vi "Handle Actor Core Events.vi"(8 "error in (no error)":errorcluster, 11 "ActorAutoRegistration":refnum<class "ActorAutoRegistration.lvclass">) -> (0 "error out":errorcluster)   [LabVIEW 2015, in "ActorEvents.lvlib" / "ActorAutoRegistration.lvclass"]
doc: "<License>\nCopyright © 2017 Composed Systems, LLC | All rights reserved\nwww.composed.io\n\nAuthor: Ethan Stern <ethan.stern@composed.io>\n\nThis software is provided \"AS IS\" WITHOUT WARRANTIES, either express or implied, AND IS FOR EDUCATIONAL PURPOSES ONLY.\n</License>"
uses:
  ActorAutoRegistration.lvclass
  ActorAutoRegistration.lvclass/ActorAutoRegistration.ctl
  IEventAggregator Messages/PanelCloseMsg/PanelCloseMsg.lvclass
  IEventAggregator Messages/ValueChangeMsg/ValueChangeMsg.lvclass
  IEventAggregator Messages/ControlMouseUpMsg/ControlMouseUpMsg.lvclass
  IEventAggregator Messages/ControlMouseDownMsg/ControlMouseDownMsg.lvclass
  IEventAggregator Messages/MenuSelectionMsg/MenuSelectionMsg.lvclass
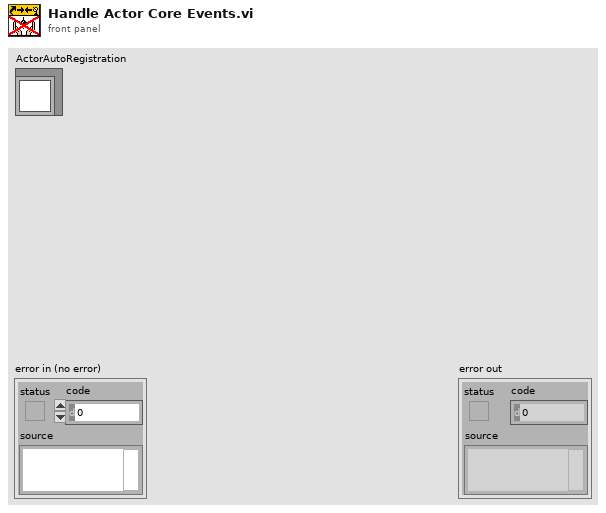
[diagram p1: front panel]
types:
  T1 = typedef "AutoRegistration.lvlib/AutoRegistration.lvclass/Auto-Event Registration Refnum.ctl" = refnum<event-registration>
  T2 = typedef "LVPoint32TypeDef.ctl" = cluster{"Horizontal":i32, "Vertical":i32}
  T3 = cluster{"Shift":bool, "Ctrl":bool, "Alt":bool, "Cmd":bool, "Opt":bool}
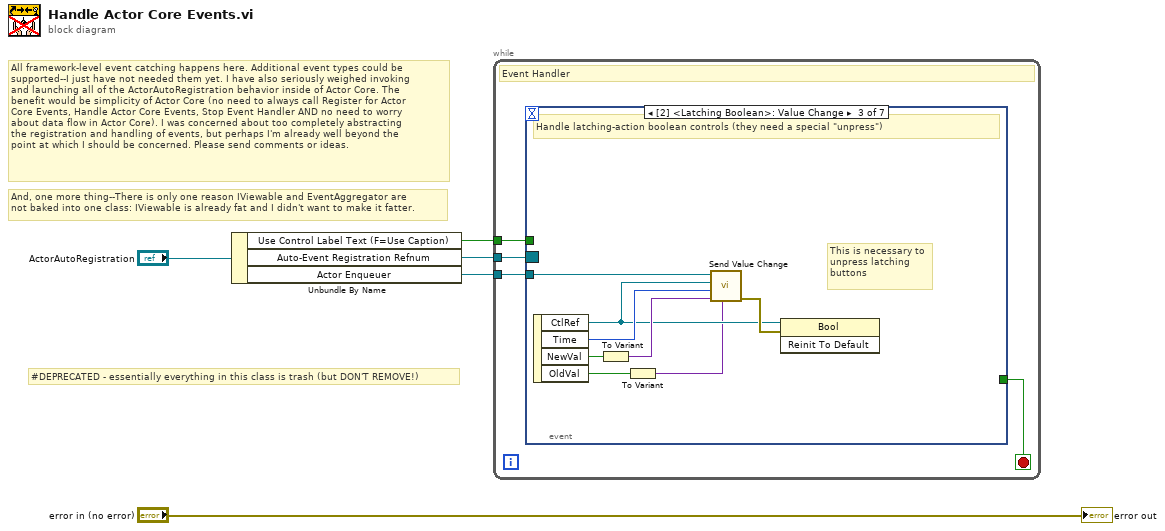
[diagram p0: block diagram]
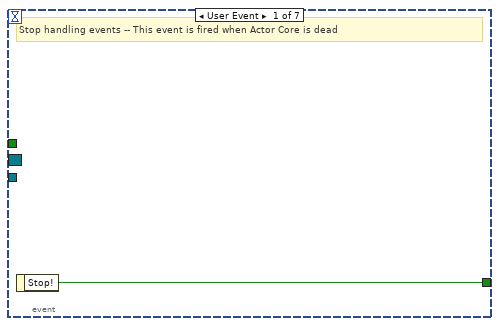
[diagram p2: hidden frame]
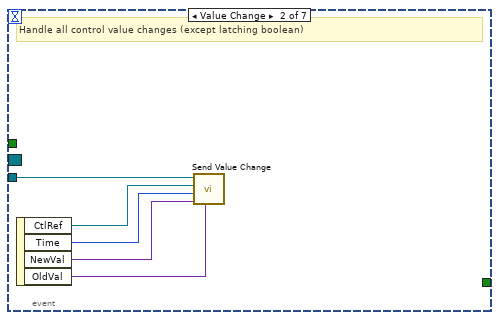
[diagram p3: hidden frame]
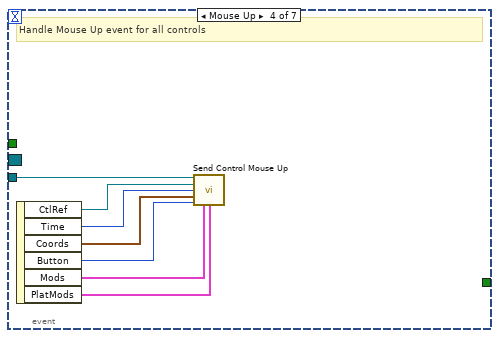
[diagram p4: hidden frame]
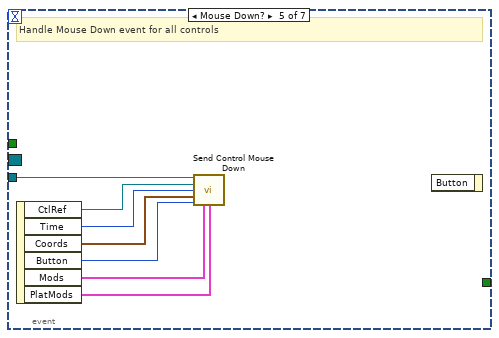
[diagram p5: hidden frame]
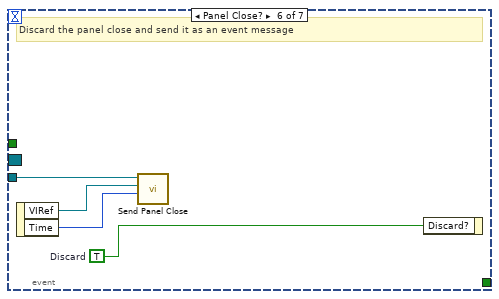
[diagram p6: hidden frame]
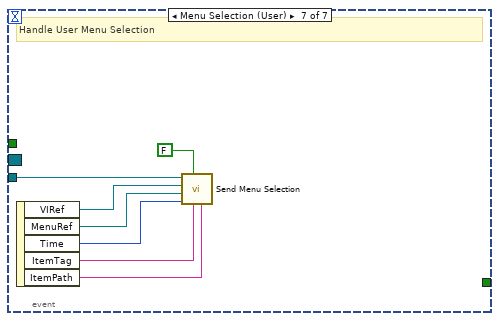
[diagram p7: hidden frame]
diagram:
  # "#DEPRECATED - essentially everything in this class is trash (but DON'T REMOVE!)"
  # "And, one more thing--There is only one reason IViewable and EventAggregator are\nnot baked into one class: IViewable is already fat and I didn't want to make it fatter."
  # "All framework-level event catching happens here. Additional event types could be\nsupported--I just have not needed them yet. I have also seriously weighed invoking\nand launching all of the ActorAutoRegistration behavior inside of Actor Core. The\nbenefit would be simplicity of Actor Core (no need to always call Register for Actor\nCore Events, Handle Actor Core Events, Stop Event Handler AND no need to worry\nabout data flow in Actor Core). I was concerned about too completely abstracting\nthe registration and handling of events, but perhaps I'm already well beyond the\npoint at which I should be concerned. Please send comments or ideas."
  n1 = Unbundle By Name("ActorAutoRegistration") -> ("Use Control Label Text (F=Use Caption)"=w2:bool, "Auto-Event Registration Refnum"=w1:T1, "Actor Enqueuer"=w3:refnum<class "Message Enqueuer.lvclass">)
  n2 = while {
    tunnel: w3 -> [w8]
    tunnel: w2 -> [w7]
    tunnel: w1 -> [w6]
    stop <- w9 stop-if-true
    # "Event Handler"
    n3 = event shown="[2] <Latching Boolean>: Value Change" {
      selector: w6 -> [_ _ _ _ _ _ _]
      dyn-events: _ -> [_ _ _ _ _ _ _]
      timeout: _ -> [_ _ _ _ _ _ _]
      tunnel: [w10 _ _ _ _ _ _] -> w9
      tunnel: w8 -> [_ w15 w23 w30 w37 w41 w48]
      tunnel: w7 -> [_ _ _ _ _ _ _]
      event User Event {
        # "Stop handling events -- This event is fired when Actor Core is dead"
        n4 = event-data() -> ("Stop!"=w10:bool)  [unwired: 1 in]
      }
      event Value Change {
        # "Handle all control value changes (except latching boolean)"
        n5 = event-data() -> ("CtlRef"=w14:refnum<vi>, "Time"=w13:u32, "NewVal"=w12:variant, "OldVal"=w11:variant)  [unwired: 1 in]
        n6 = call "Send Value Change.vi"("Old Value"=w11, "New Value"=w12, "Time"=w13, "Ctl Refnum"=w14, "Message Enqueuer in"=w15) -> ()  [unwired: 6 in, 1 out]
      }
      event Value Change {
        # "This is necessary to\nunpress latching\nbuttons"
        # "Handle latching-action boolean controls (they need a special \"unpress\")"
        n7 = event-data() -> ("CtlRef"=w18:refnum<vi>, "Time"=w20:u32, "NewVal"=w22:bool, "OldVal"=w17:bool)  [unwired: 1 in]
        n8 = To Variant(anything=w22) -> (Variant=w19:variant)
        n9 = To Variant(anything=w17) -> (Variant=w16:variant)
        n10 = call "Send Value Change.vi"("Old Value"=w16, "New Value"=w19, "Time"=w20, "Ctl Refnum"=w18, "Message Enqueuer in"=w23) -> ("error out"=w21:errorcluster)  [unwired: 6 in]
        n11 = invoke class="Bool" method="Reinit To Default"(reference=w18, error in=w21) -> ()  [unwired: 1 in, 3 out]
      }
      event Mouse Up {
        # "Handle Mouse Up event for all controls"
        n12 = event-data() -> ("CtlRef"=w29:refnum<vi>, "Time"=w28:u32, "Coords"=w27:T2, "Button"=w26:u16, "Mods"=w25:cluster{"Double Click":bool, "Menu Key":bool}, "PlatMods"=w24:T3)  [unwired: 1 in]
        n13 = call "Send Control Mouse Up.vi"("Message Enqueuer in"=w30, "Ctl Refnum"=w29, "Time"=w28, "Coords"=w27, "Button"=w26, "Mods"=w25, "PlatMods"=w24) -> ()  [unwired: 8 in, 1 out]
      }
      event Mouse Down? {
        # "Handle Mouse Down event for all controls"
        n14 = event-data() -> ("CtlRef"=w36:refnum<vi>, "Time"=w35:u32, "Coords"=w34:T2, "Button"=w33:u16, "Mods"=w32:cluster{"Double Click":bool, "Menu Key":bool}, "PlatMods"=w31:T3)  [unwired: 1 in]
        n15 = call "Send Control Mouse Down.vi"("Message Enqueuer in"=w37, "Ctl Refnum"=w36, "Time"=w35, "Coords"=w34, "Button"=w33, "Mods"=w32, "PlatMods"=w31) -> ()  [unwired: 7 in, 2 out]
        n16 = event-data() -> ()  [unwired: 2 in, 1 out]
      }
      event Panel Close? {
        w39 = TRUE  # Discard
        # "Discard the panel close and send it as an event message"
        n17 = event-data() -> ("VIRef"=w40:refnum<vi>, "Time"=w38:u32)  [unwired: 1 in]
        n18 = call "Send Panel Close.vi"("Time"=w38, "VI Refnum"=w40, "Message Enqueuer in"=w41) -> ()  [unwired: 7 in, 2 out]
        n19 = event-data("Discard?"=w39) -> ()  [unwired: 1 in, 1 out]
      }
      event Menu Selection (User) {
        # "Handle User Menu Selection"
        n20 = event-data() -> ("VIRef"=w45:refnum<vi>, "MenuRef"=w44:refnum<k9>, "Time"=w43:u32, "ItemTag"=w47:string, "ItemPath"=w46:string)  [unwired: 1 in]
        n21 = call "Send Menu Selection.vi"("Item Path"=w46, "Item Tag"=w47, "App Item?"=FALSE, "Time"=w43, "MenuRef"=w44, "VI Refnum"=w45, "Message Enqueuer in"=w48) -> ()  [unwired: 3 in, 2 out]
      }
    }
  }
  "error out" <- "error in (no error)"
